vi "addTopic.vi"(8 "error in (no error)":errorcluster, 10 "topic":string, 11 "ActiveMQBroker in":refnum<class "ActiveMQBroker.lvclass">) -> (0 "error out":errorcluster, 2 "topicID":u32, 3 "ActiveMQBroker out":refnum<class "ActiveMQBroker.lvclass">)   [LabVIEW 2012, in "ActiveMQBroker.lvclass"]
uses:
  ActiveMQBroker.lvclass
  ActiveMQBroker.lvclass/ActiveMQBroker.ctl
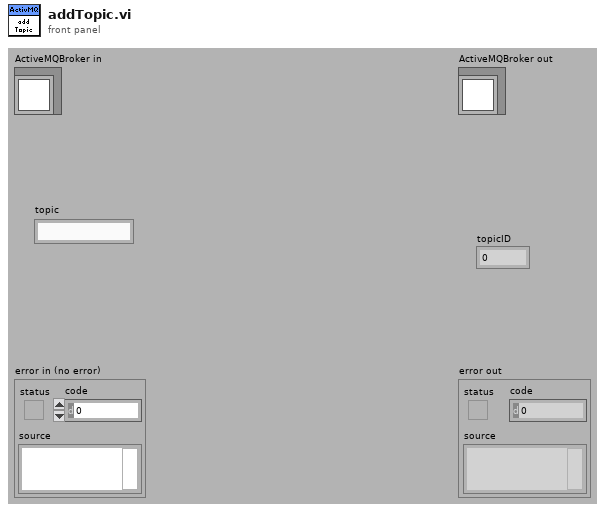
[diagram p1: front panel]
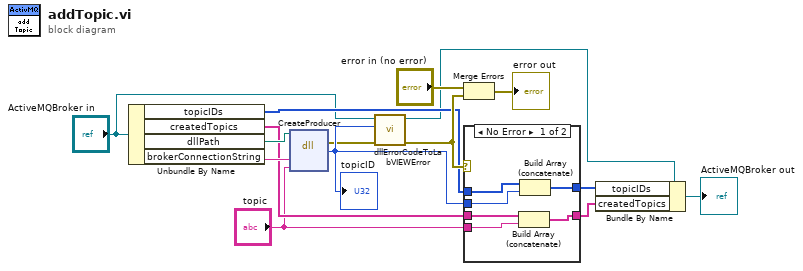
[diagram p0: block diagram]
diagram:
  n1 = Unbundle By Name("ActiveMQBroker in") -> ("topicIDs"=w3:u32[], "createdTopics"=w12:string[], "dllPath"=w15:path, "brokerConnectionString"=w14:string)
  n2 = dll-call lib="C:/Documents and Settings/dan/My Documents/Lowell/source/DCT/trunk/Components/Common/ActiveMQ/DCTActiveMQHandler/C++ Source/DCTAMQ/Release/DCTAMQ.dll" fn="CreateProducer"(path in=w15, "brokerURI"=w14, "topicName"="topic") -> (error out=w7:errorcluster, "consumerID"=w13:u32)  [unwired: 4 in, 1 out]
  "topicID" <- w13
  n3 = call "dllErrorCodeToLabVIEWError.vi"("error in (no error)"=w7, "error code in"=w13, "ActiveMQBroker in"="ActiveMQBroker in") -> ("error out"=w6:errorcluster, "ActiveMQBroker out"=w1:refnum<class "ActiveMQBroker.lvclass">)  [unwired: 7 in]
  n4 = Merge Errors("error in (no error)", w6) -> (→"error out":errorcluster)
  n5 = case shown="No Error" w6 {
    tunnel: w13 -> [w21 _]
    tunnel: w3 -> [w20 w23]
    tunnel: w12 -> [w19 w22]
    tunnel: "topic" -> [w18 _]
    tunnel: [w17 w23] -> w9
    tunnel: [w16 w22] -> w8
    frame No Error {
      n6 = Build Array (concatenate)(w19, w18) -> (w16:string[])
      n7 = Build Array (concatenate)(w20, w21) -> (w17:u32[])
    }
    frame Error {
    }
  }
  n8 = Bundle By Name(cluster=w1, "topicIDs"=w9, "createdTopics"=w8) -> (→"ActiveMQBroker out":refnum<class "ActiveMQBroker.lvclass">)
